vi "KeeperRoleVSS.vi"(6 "First call?":bool=TRUE, 8 "error in (no error)":errorcluster, 9 "Game in":refnum<class "Game.lvclass">, 10 "Robot":refnum<class "Robot.lvclass">, 11 "KeeperRoleVSS in":refnum<class "KeeperRoleVSS.lvclass">) -> (0 "error out":errorcluster, 1 "Game out":refnum<class "Game.lvclass">, 2 "Robot out":refnum<class "Robot.lvclass">, 3 "KeeperRoleVSS out":refnum<class "KeeperRoleVSS.lvclass">)   [LabVIEW 2020, in "KeeperRoleVSS.lvclass"]
uses:
  KeeperRoleVSS.lvclass
  C:/Users/lucio/Desktop/Horie/ROBOIME/VSS_AI/Role_class/Role.lvclass
  Robot_class/Robot.lvclass
  Game_class/Game.lvclass
  Role_class/Role.lvclass/Role.ctl
  Role_class/Read Tacticbook.vi
  Role_class/Read tactic_index.vi
  Role_class/Write Tacticbook.vi
  Role_class/Write tactic_index.vi
  Tacticbook_class/Tacticbook.lvclass
  DispBallTacticVSS_class/DispBallTacticVSS.lvclass
  DefendGoalTacticVSS_class/DefendGoalTacticVSS.lvclass
  PenaltyAttackTacticVSS_class/PenaltyAttackTacticVSS.lvclass
  DefendAreaTacticVSS_class/DefendAreaTacticVSS.lvclass
  AttackTacticVSS_class/AttackTacticVSS.lvclass
  HaltTactic_class/HaltTactic.lvclass
  GoAndKickTacticVSS_class/GoAndKickTacticVSS.lvclass
  GoalKickKeeperTacticVSS_class/GoalKickKeeperTacticVSS.lvclass
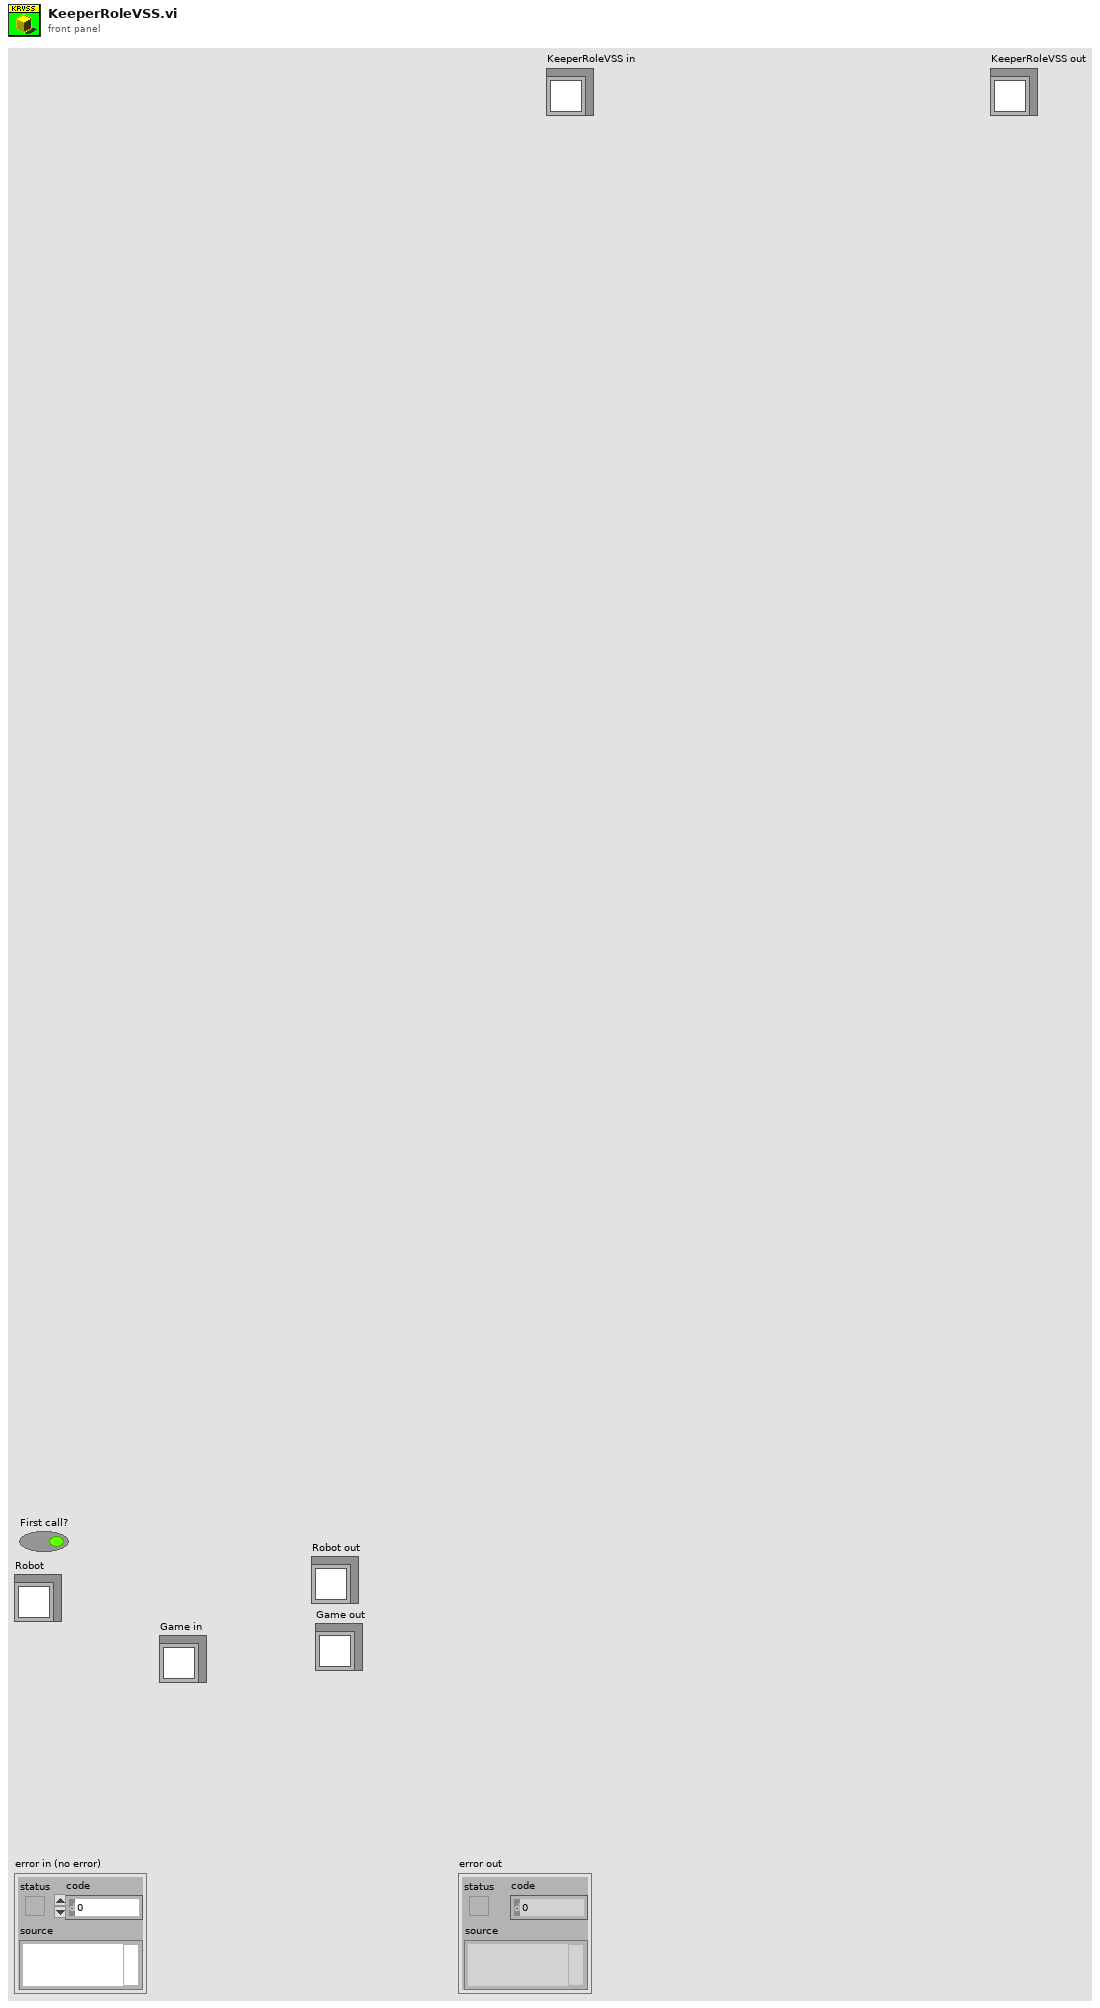
[diagram p1: front panel]
types:
  T1 = cluster{"DispBallTacticVSS":refnum<class "DispBallTacticVSS.lvclass">, "DefendGoalTacticVSS":refnum<class "DefendGoalTacticVSS.lvclass">, "PenaltyAttackTacticVSS":refnum<class "PenaltyAttackTacticVSS.lvclass">, "DefendAreaTacticVSS":refnum<class "DefendAreaTacticVSS.lvclass">, "AttackTacticVSS":refnum<class "AttackTacticVSS.lvclass">, "HaltTactic":refnum<class "HaltTactic.lvclass">, "GoAndKickTacticVSS":refnum<class "GoAndKickTacticVSS.lvclass">, "GoalKickKeeperTacticVSS":refnum<class "GoalKickKeeperTacticVSS.lvclass">}
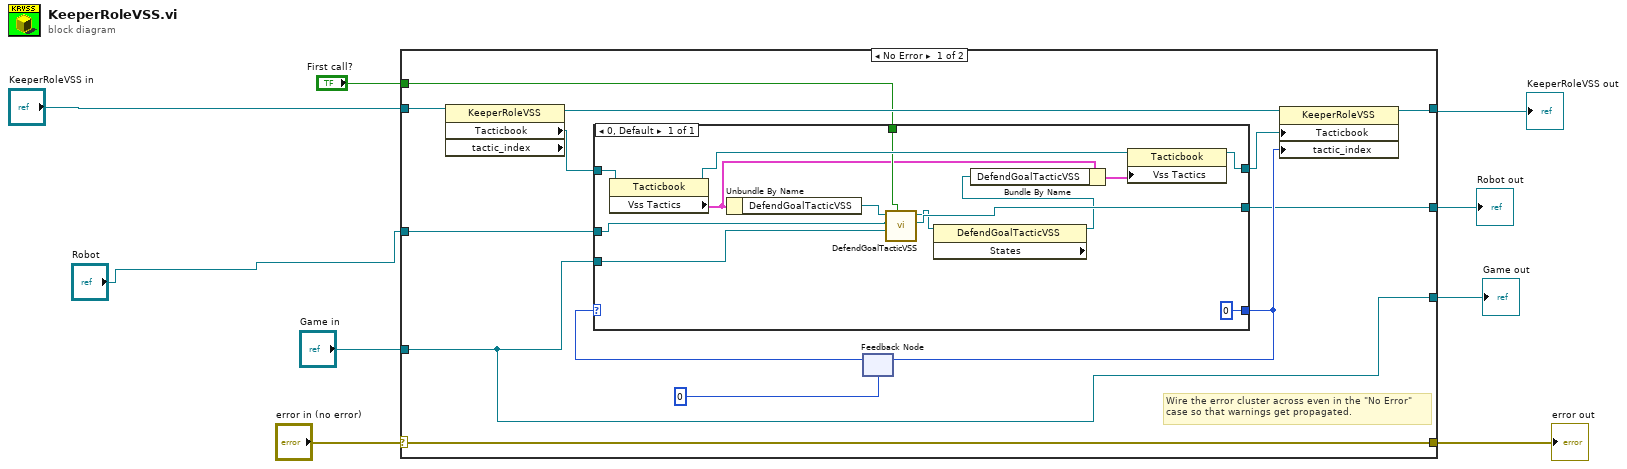
[diagram p0: block diagram]
diagram:
  n1 = case shown="No Error" "error in (no error)" {
    selector: "error in (no error)" -> [w22 w39]
    tunnel: [w22 w39] -> w8
    tunnel: [w20 w38] -> w3
    tunnel: "KeeperRoleVSS in" -> [w21 w38]
    tunnel: "Robot" -> [w14 w37]
    tunnel: [w13 w37] -> w7
    tunnel: [w11 w36] -> w6
    tunnel: "Game in" -> [w11 w36]
    tunnel: "First call?" -> [w10 _]
    frame No Error {
      # "Wire the error cluster across even in the \"No Error\"\ncase so that warnings get propagated."
      n2 = property class="KeeperRoleVSS" props=["Tacticbook", "tactic_index"](reference=w21) -> (reference out=w19:refnum<class "KeeperRoleVSS.lvclass">, "Tacticbook"=w16:refnum<class "Tacticbook.lvclass">)  [unwired: 1 in, 2 out]
      n3 = feedback #1(0) -> (w17:i32)
      n4 = case shown="0, Default" w17 {
        tunnel: [0] -> w15
        tunnel: w16 -> [w35]
        tunnel: w14 -> [w28]
        tunnel: [w30] -> w13
        tunnel: [w33] -> w12
        tunnel: w11 -> [w27]
        tunnel: w10 -> [w31]
        frame 0, Default {
          n5 = property class="Tacticbook"(reference=w35) -> (reference out=w34:refnum<class "Tacticbook.lvclass">, "Vss Tactics"=w25:T1)  [unwired: 1 in, 1 out]
          n6 = Unbundle By Name(w25) -> ("DefendGoalTacticVSS"=w26:refnum<class "DefendGoalTacticVSS.lvclass">)
          n7 = call-dynamic "DefendGoalTacticVSS.vi"("First call?"=w31, "Game in"=w27, "Robot"=w28, "DefendGoalTacticVSS in"=w26) -> ("Robot out"=w30:refnum<class "Robot.lvclass">, "DefendGoalTacticVSS out"=w29:refnum<class "DefendGoalTacticVSS.lvclass">)  [unwired: 6 in]
          n8 = property class="DefendGoalTacticVSS" props=["States"](reference=w29) -> (reference out=w23:refnum<class "DefendGoalTacticVSS.lvclass">)  [unwired: 1 in, 2 out]
          n9 = Bundle By Name(cluster=w25, "DefendGoalTacticVSS"=w23) -> (w24:T1)
          n10 = property class="Tacticbook"(reference=w34, "Vss Tactics"=w24) -> (reference out=w33:refnum<class "Tacticbook.lvclass">)  [unwired: 1 in, 1 out]
        }
      }
      n11 = feedback-in #1(w15) -> ()
      n12 = property class="KeeperRoleVSS"(reference=w19, "Tacticbook"=w12, "tactic_index"=w15) -> (reference out=w20:refnum<class "KeeperRoleVSS.lvclass">)  [unwired: 1 in, 1 out]
    }
    frame Error {
    }
  }
  "KeeperRoleVSS out" <- w3
  "error out" <- w8
  "Robot out" <- w7
  "Game out" <- w6
